vi "SetLocation.vi"(8 "error in":errorcluster, 10 "Location":string, 11 "OperationCycle in":refnum<class "OperationCycle.lvclass">) -> (0 "error out":errorcluster, 3 "OperationCycle out":refnum<class "OperationCycle.lvclass">)   [LabVIEW 2021, in "ProligentXMLGenerator.lvlib" / "OperationCycle.lvclass"]
doc: "Defines the location where the operation cycle was executed.(node/category of the full station name (site where the station is located)).\n\nThis attribute cannot be updated."
uses:
  OperationCycle.lvclass
  OperationCycle.lvclass/OperationCycle.ctl
  Base/FullName/FullName.lvclass
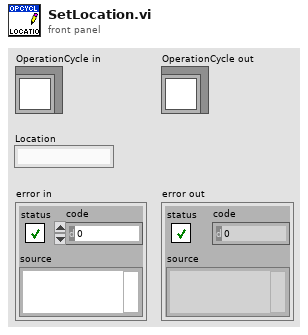
[diagram p1: front panel]
types:
  T1 = typedef "ProligentXMLGenerator.lvlib/OperationCycle.lvclass/Data.ctl" = cluster{"Name":string, "CustomData":refnum<class "CustomData.lvclass">, "ProcessFullName":refnum<class "ProcessFullName.lvclass">, "ProcessVersion":refnum<class "NonEmptyString_64.lvclass">, "OperationCycleId":refnum<class "Guid.lvclass">, "OperationName":refnum<class "NonEmptyString_65.lvclass">, "Location":refnum<class "FullName.lvclass">, "User":refnum<class "NonEmptyString_255.lvclass">, "OperationCycleStatus":refnum<class "ExecutionStatus.lvclass">, "OperationCycleStartTime":refnum<class "DateTime.lvclass">, "OperationCycleEndTime":refnum<class "DateTime.lvclass">, "TimeZoneInfoId":string}
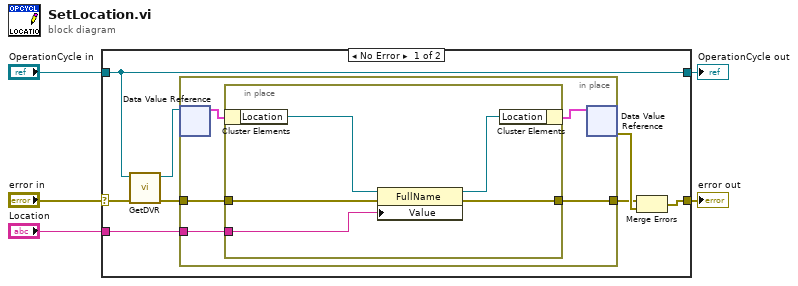
[diagram p0: block diagram]
diagram:
  n1 = case shown="No Error" "error in" {
    selector: "error in" -> [w11 w24]
    tunnel: "OperationCycle in" -> [w6 w25]
    tunnel: [w8 w24] -> w3
    tunnel: "Location" -> [w7 _]
    tunnel: [w6 w25] -> w1
    frame No Error {
      n2 = call "GetDVR.vi"("error in"=w11, "OperationCycle in"=w6) -> ("error out"=w10:errorcluster, "DVRReference"=w12:refnum<data-value>)  [unwired: 8 in]
      n3 = in-place "In Place Element Structure" {
        in-place-border: w10 -> [w18]
        in-place-border: [w16] -> w9
        in-place-border: w7 -> [w17]
        n4 = in-place-dvr #1(w12) -> (w15:T1)  [unwired: 1 out]
        n5 = in-place "In Place Element Structure" {
          in-place-border: w18 -> [w23]
          in-place-border: w17 -> [w22]
          in-place-border: [w19] -> w16
          n6 = in-place-cluster #2(w15) -> ("Location"=w21:refnum<class "FullName.lvclass">)
          n7 = property on="Property Node" class="FullName"(reference=w21, error in=w23, "Value"=w22) -> (reference out=w20:refnum<class "FullName.lvclass">, error out=w19:errorcluster)
          n8 = in-place-cluster #2("Location"=w20) -> (w14:T1)
        }
        n9 = in-place-dvr #1(w14) -> (w13:errorcluster)  [unwired: 1 out]
      }
      n10 = Merge Errors(w9, w13) -> (w8:errorcluster)
    }
    frame Error {
    }
  }
  "error out" <- w3
  "OperationCycle out" <- w1
